vi "Hex-bt.vi"() -> ()   [LabVIEW 2012]
uses:
  <vilib>/Instr/_visa.llb/VISA Set IO Buffer Mask.ctl
  <vilib>/Instr/_visa.llb/VISA Configure Serial Port (Instr).vi
panel:
  out "Tank":u8(slide) scale=0.0..5.0
  out "String":string
  in  "Right":bool
  in  "Lift":i16(knob)=20 min=-50 max=77 step=1 scale=-50.0..77.0
  in  "Turn":i16(knob)=20 min=-30 max=30 step=1 scale=30.0..-30.0
  in  "Connection settings":enum32{"Simple", "Advanced"}(tab)
  in  "VISA resource name":refnum<visa-resource-name>
  in  "baud rate (9600)":u32=9600
  in  "Mask":T1=16 items=["I/O Receive Buffer"=16, "I/O Transmit Buffer"=32, "I/O Receive and Transmit Buffer"=48]
  in  "data bits (8)":u16=8 min=5 max=8 step=1
  in  "parity (0:none)":enum16{"None", "Odd", "Even", "Mark", "Space"}(ring)
  in  "stop bits (10: 1 bit)":u16(ring)=10 items=["1.0"=10, "1.5"=15, "2.0"=20]
  in  "Left":bool
  in  "POWER":bool
  in  "Speed":u8(slide)=1 min=1 max=10 step=1 scale=1.0..10.0
  in  "Back":bool
  in  "Forth":bool
  in  "Mode":u8(slide) max=1 step=1 scale=0.0..1.0
  in  "stop":bool
  in  "LEG4":bool
  in  "LEG3":bool
  in  "LEG5":bool
  in  "LEG2":bool
  in  "LEG6":bool
  in  "LEG1":bool
  out "return count":u32
  out "write \nreturn count":u32
  out "read buffer":string
  # "Auto"
  # "Manual"
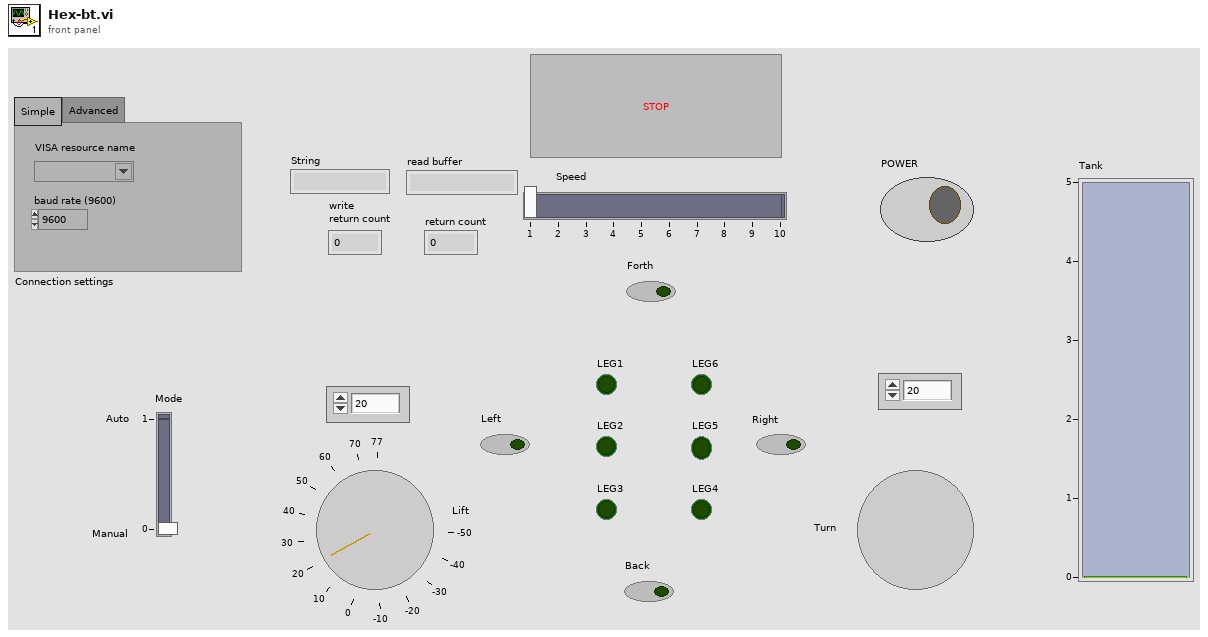
[diagram p1: front panel]
types:
  T1 = typedef "VISA Set IO Buffer Mask.ctl" = u16
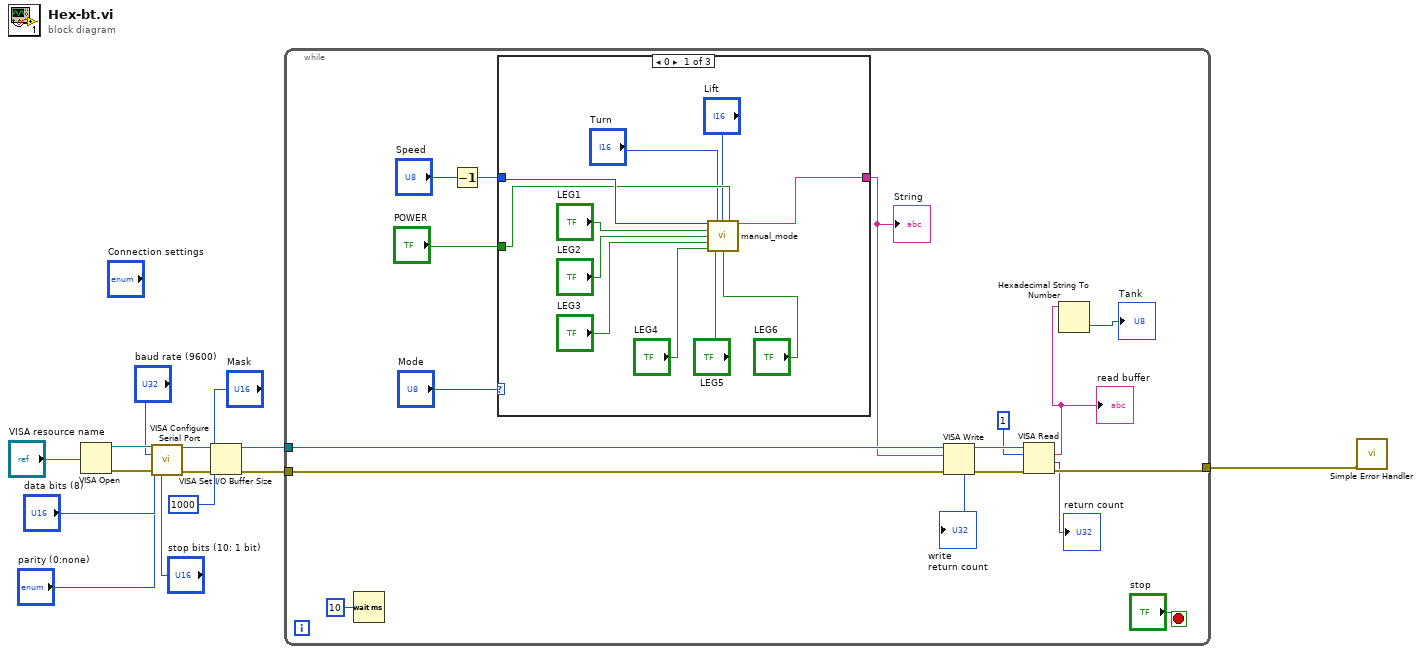
[diagram p0: block diagram]
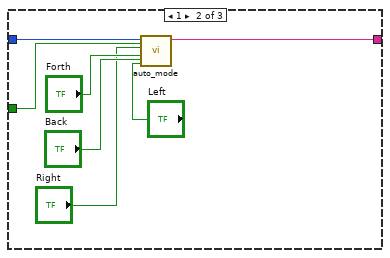
[diagram p2: hidden frame]
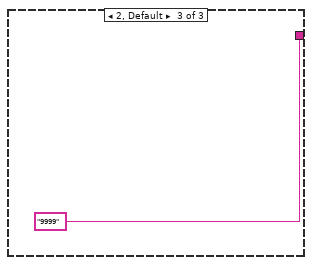
[diagram p3: hidden frame]
diagram:
  n1 = VISA Open(VISA resource name="VISA resource name") -> (VISA resource name=w13:refnum<visa-resource-name>, error out=w12:errorcluster)  [unwired: 4 in]
  n2 = call-poly "VISA Configure Serial Port"("VISA resource name"=w13, "baud rate (9600)"="baud rate (9600)", "data bits (8)"="data bits (8)", "parity (0:none)"="parity (0:none)", "error in (no error)"=w12, "stop bits (10: 1 bit)"="stop bits (10: 1 bit)") -> ("VISA resource name out"=w7:refnum<visa-resource-name>, "error out"=w4:errorcluster)  [unwired: 8 in]
  n3 = VISA Set I/O Buffer Size(VISA resource name=w7, mask (16)="Mask", size (4096)=u32 1000, error in (no error)=w4) -> (VISA resource name out=w6:refnum<visa-resource-name>, error out=w5:errorcluster)
  n4 = while {
    tunnel: w6 -> [w30]
    tunnel: w5 -> [w29]
    tunnel: [w21] -> w1
    stop <- "stop" stop-if-true
    n5 = Wait (ms)(milliseconds to wait=u32 10) -> ()  [unwired: 1 out]
    n6 = Decrement(x="Speed") -> (x-1=w22:u8)
    n7 = case shown="0" "Mode" {
      tunnel: [w42 w49 "9999"] -> w24
      tunnel: w22 -> [w41 w45 _]
      tunnel: "POWER" -> [w34 w44 _]
      frame 0 {
        n8 = call "manual_mode.vi"("Speed"=w41, "Turn"="Turn", "Lift"="Lift", "POWER"=w34, "LEG1"="LEG1", "LEG2"="LEG2", "LEG3"="LEG3", "LEG4"="LEG4", "LEG5"="LEG5", "LEG6"="LEG6") -> ("String"=w42:string)  [unwired: 5 in]
      }
      frame 1 {
        n9 = call "auto_mode.vi"("Back"="Back", "POWER"=w44, "Left"="Left", "Forth"="Forth", "Right"="Right", "Speed"=w45) -> ("String"=w49:string)  [unwired: 5 in]
      }
      frame 2, Default {
      }
    }
    "String" <- w24
    n10 = VISA Write(VISA resource name=w30, write buffer=w24, error in (no error)=w29) -> (VISA resource name out=w19:refnum<visa-resource-name>, return count=→"write \nreturn count":u32, error out=w20:errorcluster)
    n11 = VISA Read(VISA resource name=w19, byte count=u32 1, error in (no error)=w20) -> (read buffer=w15:string, return count=→"return count":u32, error out=w21:errorcluster)  [unwired: 1 out]
    "read buffer" <- w15
    n12 = Hexadecimal String To Number(string=w15) -> (number=→"Tank":u32)  [unwired: 2 in, 1 out]
  }
  n13 = call <vilib>:"Simple Error Handler.vi"("error in (no error)"=w1) -> ()  [unwired: 4 in, 5 out]
